vi "Elevator Object Counter.vi"(5 "Clear Stack?":bool, 7 "Toggle Trashcan?":bool, 8 "Trashcan Delta":i32, 10 "Tote Delta":i32) -> (0 "Have Trashcan":bool, 2 "Tote Count":i8)   [LabVIEW 2014]
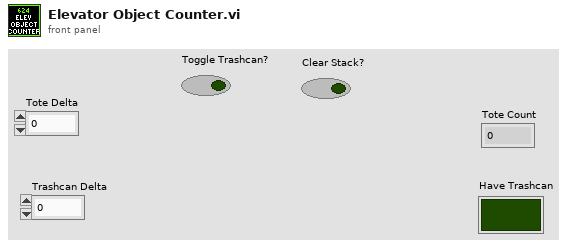
[diagram p1: front panel]
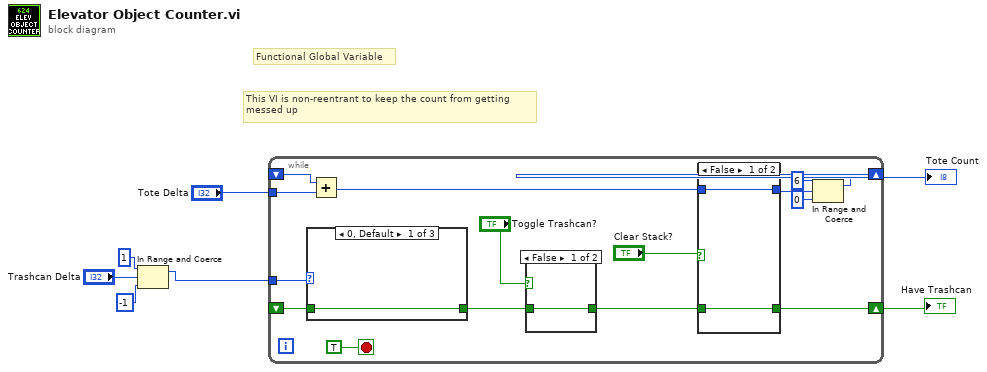
[diagram p0: block diagram]
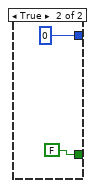
[diagram p2: hidden frame]
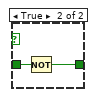
[diagram p3: hidden frame]
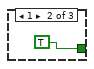
[diagram p4: hidden frame]
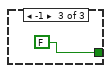
[diagram p5: hidden frame]
diagram:
  # "Functional Global Variable"
  # "This VI is non-reentrant to keep the count from getting\nmessed up"
  n1 = In Range and Coerce(upper limit=1, x="Trashcan Delta", lower limit=-1) -> (coerced(x)=w2:i32)  [unwired: 1 out]
  n2 = while {
    shift-right: [w13] -> w1
    shift-left: _ -> [w18]
    shift-right: [w8] -> w7
    shift-left: _ -> [w21]
    tunnel: "Tote Delta" -> [w20]
    tunnel: w2 -> [w19]
    stop <- TRUE stop-if-true
    n3 = case shown="0, Default" w19 {
      tunnel: [w30 TRUE FALSE] -> w16
      tunnel: w18 -> [w30 _ _]
      frame 0, Default {
      }
      frame 1 {
      }
      frame -1 {
      }
    }
    n4 = Add(x=w21, y=w20) -> (x+y=w12:i32)
    n5 = case shown="False" "Toggle Trashcan?" {
      tunnel: w16 -> [w27 w29]
      tunnel: [w27 w28] -> w14
      frame False {
      }
      frame True {
        n6 = Not(x=w29) -> (.not. x?=w28:bool)
      }
    }
    n7 = case shown="False" "Clear Stack?" {
      tunnel: w14 -> [w23 _]
      tunnel: [w23 FALSE] -> w13
      tunnel: [w24 0] -> w11
      tunnel: w12 -> [w24 _]
      frame False {
      }
      frame True {
      }
    }
    n8 = In Range and Coerce(upper limit=6, x=w11, lower limit=0) -> (coerced(x)=w8:i32)  [unwired: 1 out]
  }
  "Have Trashcan" <- w1
  "Tote Count" <- w7
